vi "GETPINSTATUS.vi"(8 "error in (no error)":errorcluster, 9 "pin":dbl, 10 "Port":dbl, 11 "NXP in":refnum<class "NXP.lvclass">) -> (0 "error out":errorcluster, 3 "NXP out":refnum<class "NXP.lvclass">)   [LabVIEW 2019, in "NXP.lvclass"]
uses:
  NXP.lvclass
  NXP.lvclass/NXP.ctl
  ac2fb357-8850-47d5-8f3c-7eeb2fb3dcfd.vi
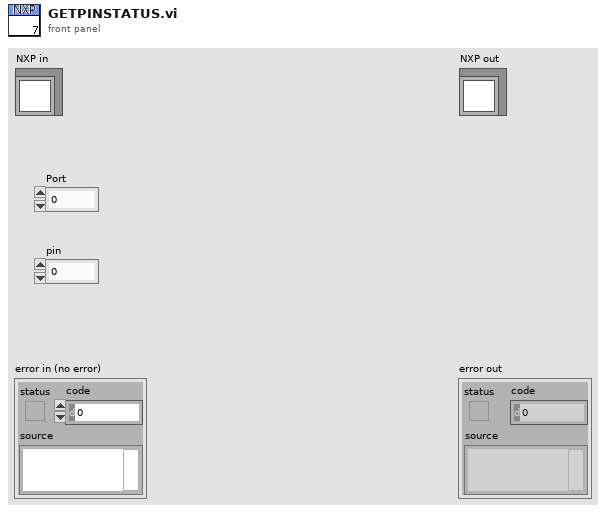
[diagram p1: front panel]
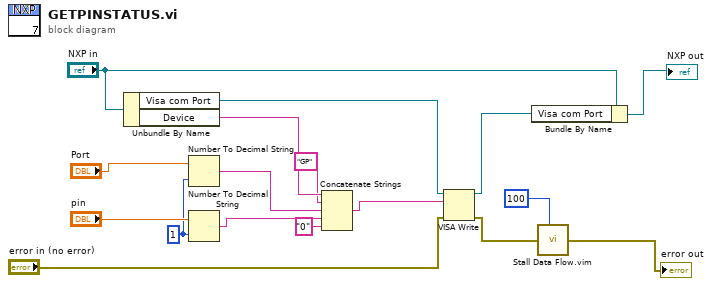
[diagram p0: block diagram]
diagram:
  w15 = i16 1 ("width (-)")
  n1 = Unbundle By Name("NXP in") -> ("Visa com Port"=w12:refnum<visa-resource-name>, "Device"=w14:string)
  n2 = Number To Decimal String(number="Port", width (-)=w15) -> (decimal integer string=w10:string)
  n3 = Number To Decimal String(number="pin", width (-)=w15) -> (decimal integer string=w9:string)
  n4 = Concatenate Strings(w14, "GP" ("string"), w10, w9, "0" ("string")) -> (w13:string)
  n5 = VISA Write(VISA resource name=w12, write buffer=w13, error in (no error)="error in (no error)") -> (VISA resource name out=w1:refnum<visa-resource-name>, error out=w7:errorcluster)  [unwired: 1 out]
  n6 = Bundle By Name(cluster="NXP in", "Visa com Port"=w1) -> (→"NXP out":refnum<class "NXP.lvclass">)
  n7 = call "Stall Data Flow.vim"("value in"=w7, "milliseconds to wait"=u32 100) -> ("value out"=→"error out":errorcluster)  [unwired: 1 out]
